vi "Read Element of Array - Numeric.vi"(8 "error in (no error)":errorcluster, 10 "index":i32, 11 "TAS_Message in":refnum<class "TAS_Message.lvclass">) -> (0 "error out":errorcluster, 2 "Numeric":dbl, 3 "TAS_Message out":refnum<class "TAS_Message.lvclass">)   [LabVIEW 2012, in "TAS_Message.lvclass"]
uses:
  TAS_Message.lvclass
  TAS_Message.lvclass/TAS_Message.ctl
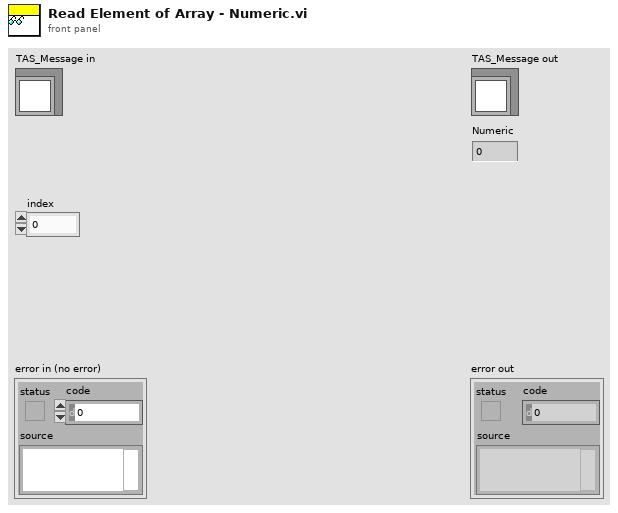
[diagram p1: front panel]
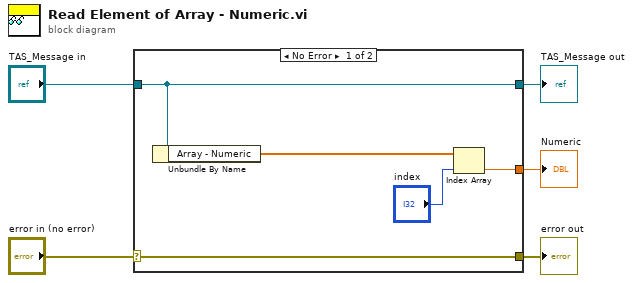
[diagram p0: block diagram]
diagram:
  n1 = case shown="No Error" "error in (no error)" {
    selector: "error in (no error)" -> [w10 w11]
    tunnel: [w10 w11] -> w4
    tunnel: [w9 w12] -> w2
    tunnel: "TAS_Message in" -> [w9 w12]
    tunnel: [w6 _] -> w1
    frame No Error {
      n2 = Unbundle By Name(w9) -> ("Array - Numeric"=w8:dbl[])
      n3 = Index Array(array=w8, index="index") -> (element=w6:dbl)
    }
    frame Error {
    }
  }
  "error out" <- w4
  "TAS_Message out" <- w2
  "Numeric" <- w1
